vi "Write myClass3Array.vi"(8 "error in (no error)":errorcluster, 10 "class3Array":refnum<class "Class3.lvclass">[](array[class]), 11 "Test1 in":refnum<class "Class1.lvclass">) -> (0 "error out":errorcluster, 3 "Test1 out":refnum<class "Class1.lvclass">)   [LabVIEW 2020, in "Class1.lvclass"]
doc: "GCraftsman JSON Object Serialization Toolkit\nwww.GCraftsman.com\nCopyright (c) 2017, GCraftsman"
uses:
  Class1.lvclass
  Class1.lvclass/Class1.ctl
  Class3/Class3.lvclass
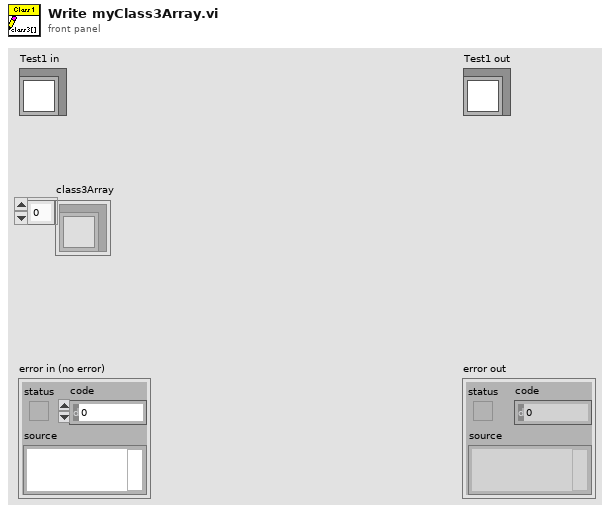
[diagram p1: front panel]
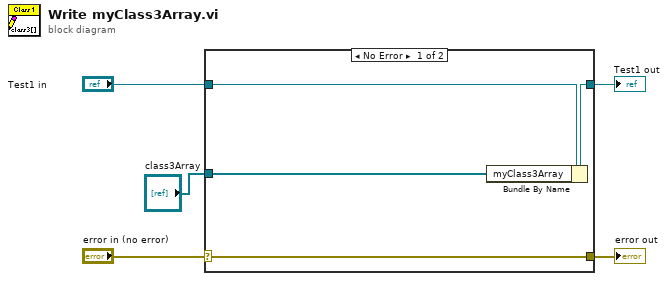
[diagram p0: block diagram]
diagram:
  n1 = case shown="No Error" "error in (no error)" {
    selector: "error in (no error)" -> [w9 w10]
    tunnel: [w9 w10] -> w4
    tunnel: [w7 w11] -> w2
    tunnel: "Test1 in" -> [w8 w11]
    tunnel: "class3Array" -> [w6 _]
    frame No Error {
      n2 = Bundle By Name(cluster=w8, "myClass3Array"=w6) -> (w7:refnum<class "Class1.lvclass">)
    }
    frame Error {
    }
  }
  "error out" <- w4
  "Test1 out" <- w2
